vi "CT_BuildError.vi"(9 "New Error":errorcluster, 10 "Error Array In":errorcluster[](array[cluster])) -> (2 "Error Array Out":errorcluster[](array[cluster]))   [LabVIEW 2020]
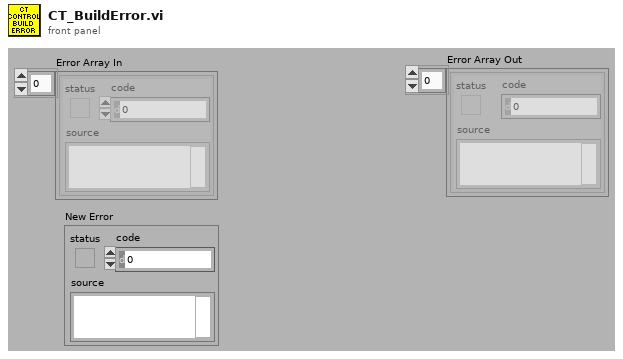
[diagram p1: front panel]
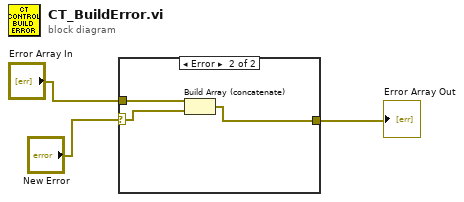
[diagram p0: block diagram]
diagram:
  n1 = case shown="Error" "New Error" {
    selector: "New Error" -> [_ w7]
    tunnel: [w4 w6] -> w1
    tunnel: "Error Array In" -> [w4 w5]
    frame No Error {
    }
    frame Error {
      n2 = Build Array (concatenate)(w5, w7) -> (w6:errorcluster[])
    }
  }
  "Error Array Out" <- w1
